vi "NI OCR-Search Ctl Reference By Label.vi"(8 "error in":errorcluster, 10 "Ctl Label":string, 11 "Buffer Data In":T1={"VI Refnum"=refnum, "Src Image"=refnum, "Dst Image"=refnum, "Ctl Refnum []"=[], "Ctl Label"=[], "User Event"=refnum, "Event Registration Refnum"=refnum, "Timeout"=0, "IMAQ OCR Session"=refnum, "Objects"=[], "ROI Descriptor"={"Global Rectangle"=[], "Contours"=[]}, "Settings"={"Objects"=0, "Threshold"=128, "Reject Border"=FALSE, "Fill Holes"=FALSE, "Min Object Size"=FALSE, "Min Size"=3, "Max Object Size"=FALSE, "Max Size"=100, "Show Search Area"=FALSE, "Show Center"=TRUE, "Show Bounding Box"=TRUE}} {"Settings"."Objects" items=["Bright Objects", "Dark Objects"]; "Settings"."Threshold" min=1 max=999999999 step=1; "Settings"."Max Size" min=1 max=999999999 step=1; "Settings"."Min Size" min=1 max=999999999 step=1; "ROI Descriptor"."Contours"."Type" items=["No Selection", "Point", "Line", "Rectangle", "Oval", "Polygon", "Freehand Region", "Annulus", "Unused2", "Unused3", "Broken Line", "Freehand Line", "Rotated Rectangle"]; "Objects"."Aspect Ratio" format="%.2f"; "Objects"."Orientation" format="%.2f"; "Objects"."Area" format="%.2f"; "Objects"."Object Center"."Y" format="%.2f"; "Objects"."Object Center"."X" format="%.2f"}) -> (0 "error out":errorcluster, 1 "Find?":bool, 2 "Ctl Refnum":refnum<vi>, 3 "Buffer Data Out":T1={"VI Refnum"=refnum, "Src Image"=refnum, "Dst Image"=refnum, "Ctl Refnum []"=[], "Ctl Label"=[], "User Event"=refnum, "Event Registration Refnum"=refnum, "Timeout"=0, "IMAQ OCR Session"=refnum, "Objects"=[], "ROI Descriptor"={"Global Rectangle"=[], "Contours"=[]}, "Settings"={"Objects"=0, "Threshold"=128, "Reject Border"=FALSE, "Fill Holes"=FALSE, "Min Object Size"=FALSE, "Min Size"=3, "Max Object Size"=FALSE, "Max Size"=100, "Show Search Area"=FALSE, "Show Center"=TRUE, "Show Bounding Box"=TRUE}} {"Settings"."Objects" items=["Bright Objects", "Dark Objects"]; "Settings"."Threshold" min=1 max=999999999 step=1; "Settings"."Max Size" min=1 max=999999999 step=1; "Settings"."Min Size" min=1 max=999999999 step=1; "ROI Descriptor"."Contours"."Type" items=["No Selection", "Point", "Line", "Rectangle", "Oval", "Polygon", "Freehand Region", "Annulus", "Unused2", "Unused3", "Broken Line", "Freehand Line", "Rotated Rectangle"]; "Objects"."Aspect Ratio" format="%.2f"; "Objects"."Orientation" format="%.2f"; "Objects"."Area" format="%.2f"; "Objects"."Object Center"."Y" format="%.2f"; "Objects"."Object Center"."X" format="%.2f"})   [LabVIEW 2016]
uses:
  Data Def/NI OCR-Buffer Data.ctl
  <vilib>/vision/Image Controls.llb/IMAQ Image.ctl
  Data Def/NI OCR-User Event Data.ctl
  <vilib>/vision/OCR.llb/IMAQ OCR Session.ctl
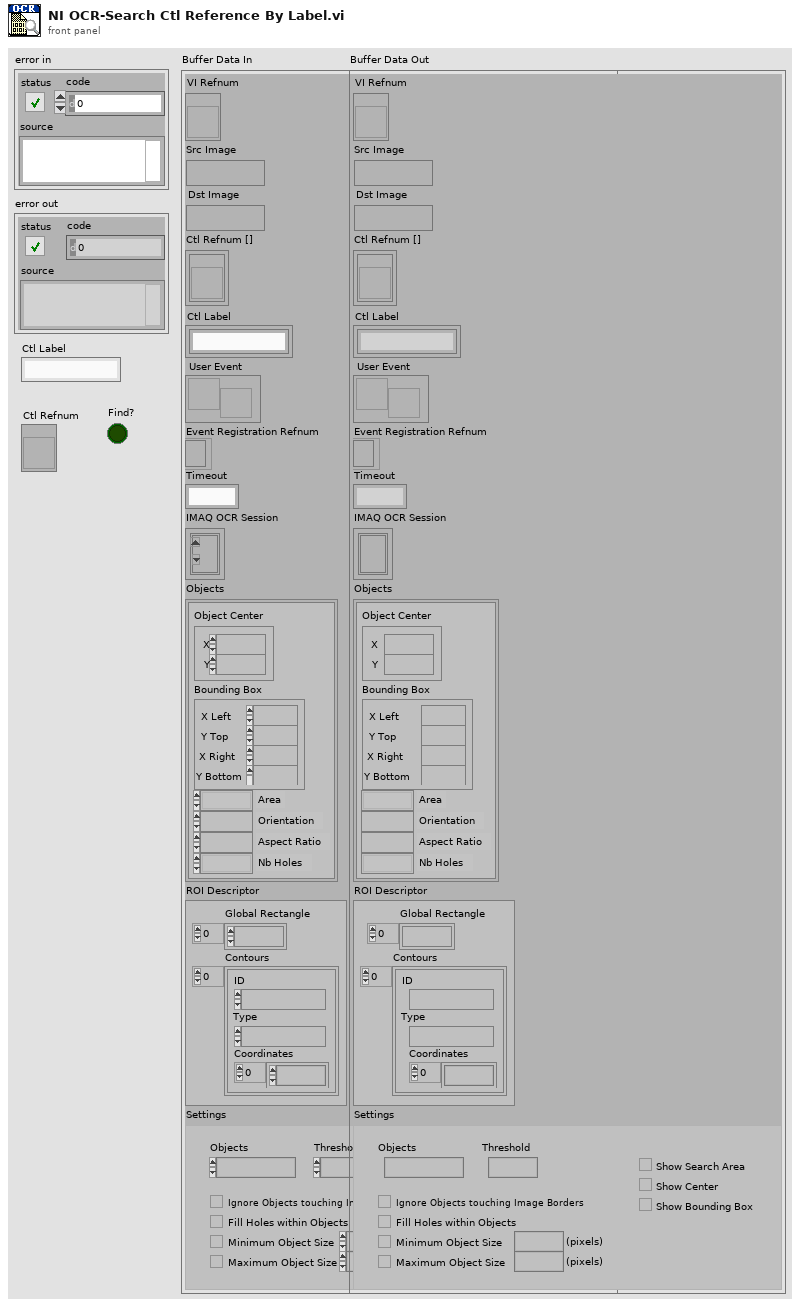
[diagram p1: front panel]
types:
  T1 = typedef "NI OCR-Buffer Data.ctl" = cluster{"VI Refnum":refnum<vi>, "Src Image":T2, "Dst Image":T2, "Ctl Refnum []":refnum<vi>[], "Ctl Label":string[], "User Event":refnum<user-event>, "Event Registration Refnum":refnum<event-registration>, "Timeout":i32, "IMAQ OCR Session":T3, "Objects":cluster{"Object Center":cluster{"X":sgl, "Y":sgl}, "Bounding Box":cluster{"X Left":i32, "Y Top":i32, "X Right":i32, "Y Bottom":i32}, "Area":sgl, "Orientation":sgl, "Aspect Ratio":sgl, "Nb Holes":i32}[], "ROI Descriptor":T4, "Settings":cluster{"Objects":u16, "Threshold":i32, "Reject Border":bool, "Fill Holes":bool, "Min Object Size":bool, "Min Size":i32, "Max Object Size":bool, "Max Size":i32, "Show Search Area":bool, "Show Center":bool, "Show Bounding Box":bool}}
  T2 = typedef "IMAQ Image.ctl" = refnum<image>
  T3 = typedef "IMAQ OCR Session.ctl" = refnum<k1>
  T4 = typedef "ROI Descriptor" = cluster{"Global Rectangle":i32[], "Contours":cluster{"ID":enum32{"External", "Internal"}, "Type":u32, "Coordinates":i32[]}[]}
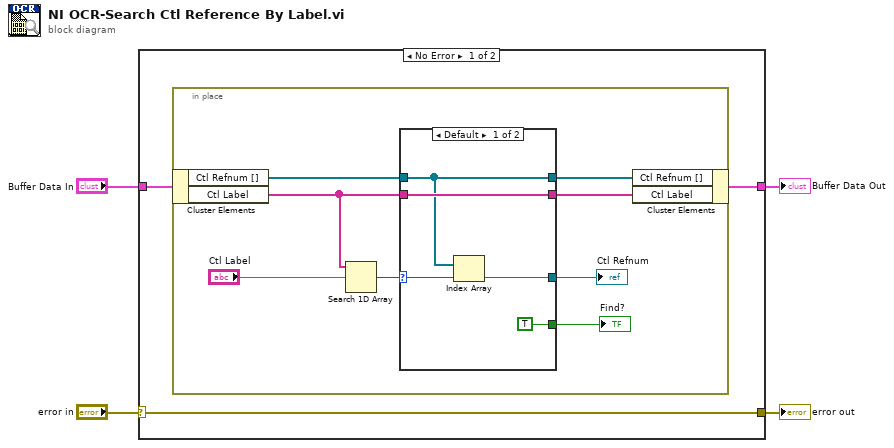
[diagram p0: block diagram]
diagram:
  n1 = case shown="No Error" "error in" {
    selector: "error in" -> [w5 w24]
    tunnel: "Buffer Data In" -> [w7 w23]
    tunnel: [w6 w23] -> w3
    tunnel: [w5 w24] -> w1
    frame No Error {
      n2 = in-place {
        n3 = in-place-cluster #1(w7) -> ("Ctl Refnum []"=w14:refnum<vi>[], "Ctl Label"=w13:string[])
        n4 = Search 1D Array(1D array=w13, element="Ctl Label") -> (index of element=w12:i32)  [unwired: 1 in]
        n5 = case shown="Default" w12 {
          selector: w12 -> [w19 _]
          tunnel: w14 -> [w18 w21]
          tunnel: w13 -> [w20 w22]
          tunnel: [w20 w22] -> w11
          tunnel: [w18 w21] -> w10
          tunnel: [w17 _] -> w9
          tunnel: [TRUE _] -> w8
          frame Default {
            n6 = Index Array(array=w18, index=w19) -> (element=w17:refnum<vi>)
          }
          frame -1 {
          }
        }
        "Ctl Refnum" <- w9
        "Find?" <- w8
        n7 = in-place-cluster #1("Ctl Refnum []"=w10, "Ctl Label"=w11) -> (w6:T1)
      }
    }
    frame Error {
    }
  }
  "error out" <- w1
  "Buffer Data Out" <- w3
